vi "get TED_Status.vi"(8 "error in (no error)":errorcluster, 11 "TED-VISA In":refnum<visa-resource-name> caption="instrument handle") -> (0 "error out":errorcluster, 2 "TED Status":T1, 3 "TED-VISA Out":refnum<visa-resource-name> caption="instrument handle out")   [LabVIEW 2025]
doc: "Use this template to build a VI to use as a subVI."
uses:
  controls/TED4015 Status.ctl
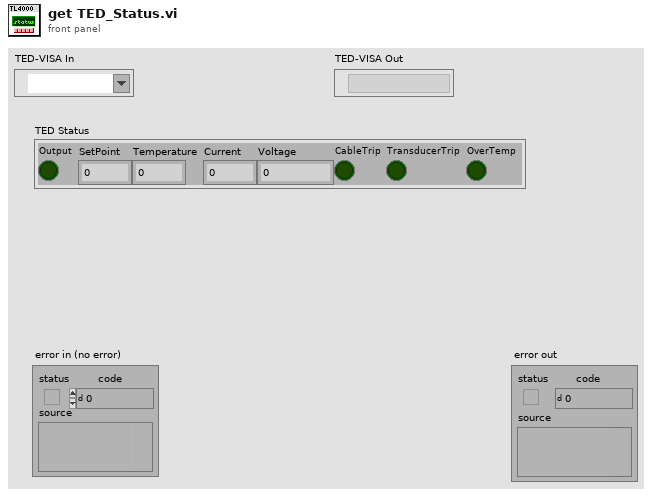
[diagram p1: front panel]
types:
  T1 = typedef "TED4015 Status.ctl" = cluster{"Output":bool, "SetPoint":dbl, "Temperature":dbl, "Current":dbl, "Voltage":dbl, "CableTrip":bool, "TransducerTrip":bool, "OverTemp":bool}
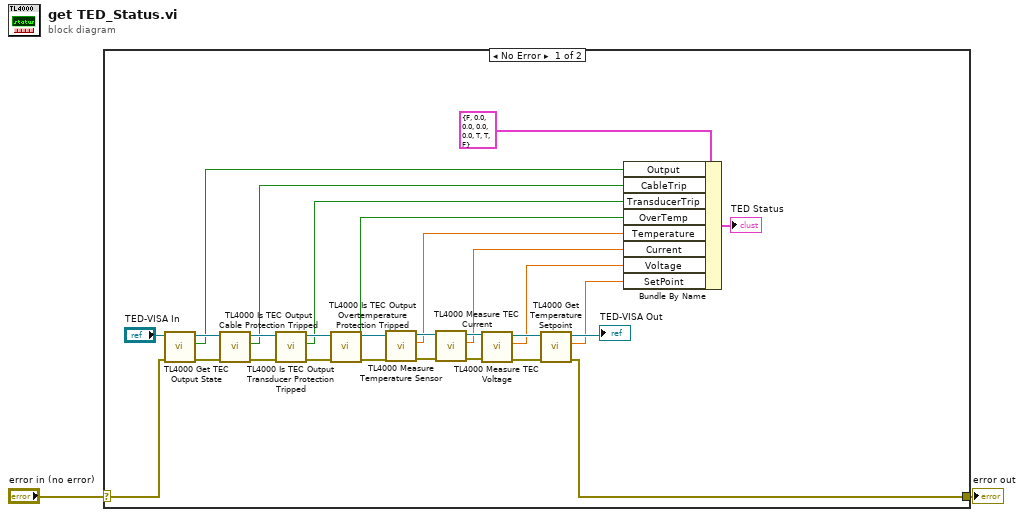
[diagram p0: block diagram]
diagram:
  n1 = case shown="No Error" "error in (no error)" {
    selector: "error in (no error)" -> [w23 w31]
    tunnel: [w16 w31] -> w1
    frame No Error {
      n2 = call <instrlib>:"TL4000 Get TEC Output State.vi"("error in (no error)"=w23, "instrument handle"="TED-VISA In") -> ("error out"=w28:errorcluster, "TEC Output"=w11:bool, "instrument handle out"=w26:refnum<visa-resource-name>)  [unwired: 7 in]
      n3 = call <instrlib>:"TL4000 Is TEC Output Cable Protection Tripped.vi"("error in (no error)"=w28, "instrument handle"=w26) -> ("error out"=w27:errorcluster, "Tripped"=w10:bool, "instrument handle out"=w25:refnum<visa-resource-name>)  [unwired: 7 in]
      n4 = call <instrlib>:"TL4000 Is TEC Output Transducer Protection Tripped.vi"("error in (no error)"=w27, "instrument handle"=w25) -> ("error out"=w30:errorcluster, "Tripped"=w9:bool, "instrument handle out"=w29:refnum<visa-resource-name>)  [unwired: 7 in]
      n5 = call <instrlib>:"TL4000 Is TEC Output Overtemperature Protection Tripped.vi"("error in (no error)"=w30, "instrument handle"=w29) -> ("error out"=w15:errorcluster, "Tripped"=w8:bool, "instrument handle out"=w14:refnum<visa-resource-name>)  [unwired: 7 in]
      n6 = call <instrlib>:"TL4000 Measure Temperature Sensor.vi"("error in (no error)"=w15, "instrument handle"=w14) -> ("error out"=w22:errorcluster, "Temperature Sensor Signal"=w7:dbl, "instrument handle out"=w21:refnum<visa-resource-name>)  [unwired: 7 in]
      n7 = call <instrlib>:"TL4000 Measure TEC Current.vi"("error in (no error)"=w22, "instrument handle"=w21) -> ("error out"=w20:errorcluster, "TEC Current"=w6:dbl, "instrument handle out"=w19:refnum<visa-resource-name>)  [unwired: 7 in]
      n8 = call <instrlib>:"TL4000 Measure TEC Voltage.vi"("error in (no error)"=w20, "instrument handle"=w19) -> ("error out"=w18:errorcluster, "TEC Voltage"=w5:dbl, "instrument handle out"=w17:refnum<visa-resource-name>)  [unwired: 7 in]
      n9 = call <instrlib>:"TL4000 Get Temperature Setpoint.vi"("error in (no error)"=w18, "instrument handle"=w17) -> ("error out"=w16:errorcluster, "Temperature Setpoint"=w4:dbl, "instrument handle out"=→"TED-VISA Out":refnum<visa-resource-name>)  [unwired: 7 in]
      n10 = Bundle By Name(cluster=T1 {"Output"=FALSE, "SetPoint"=0.0, "Temperature"=0.0, "Current"=0.0, "Voltage"=0.0, "CableTrip"=TRUE, "TransducerTrip"=TRUE, "OverTemp"=FALSE} ("TedStatus"), "Output"=w11, "CableTrip"=w10, "TransducerTrip"=w9, "OverTemp"=w8, "Temperature"=w7, "Current"=w6, "Voltage"=w5, "SetPoint"=w4) -> (→"TED Status":T1)
    }
    frame Error {
    }
  }
  "error out" <- w1
